vi "PI_GCS3_Configuration_Setup_FRF.vi"(0 "System no.":i32=1 min=1 step=1, 1 "Conn. Axes":string[](array[string]), 3 "Reference mode":enum16{"Do not reference", "Reference switch"}[](array[ring]), 5 "error in":errorcluster, 7 "Stop refnum":refnum<vi>) -> (19 "error out":errorcluster)   [LabVIEW 2020]
doc: "Select axes which reference mode is not \"Do not reference\" and waits until referenced with FRF. Former GCS 2.0 commands FPL/FNL are not supported any more.\n\nWarning: Do not use this VI outside the GCS 3.0 Configuration Setup."
uses:
  Special command.llb/ModeOfOperation.ctl
panel:
  # "Select axes which reference mode is not\n\"Do not reference\" and waits until referenced\nwith FRF. Former GCS 2.0 commands FPL/FNL\nare not supported any more.\n\nWarning: Do not use this VI outside the\nGCS 3.0 Configuration Setup."
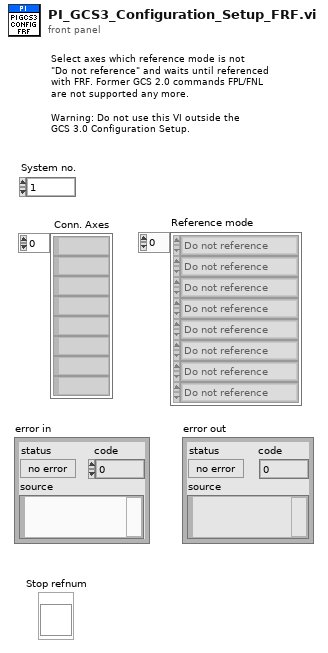
[diagram p1: front panel]
types:
  T1 = typedef "ModeOfOperation.ctl" = enum16{"Open", "Open-Loop Position", "Closed-Loop Position", "Open-Loop Velocity", "Closed-Loop Velocity", "Open-Loop Force", "Closed-Loop Force", "Step Operation"}
  T2 = typedef "Status.ctl" = cluster{"Element":string, "Status bits":bool[]}
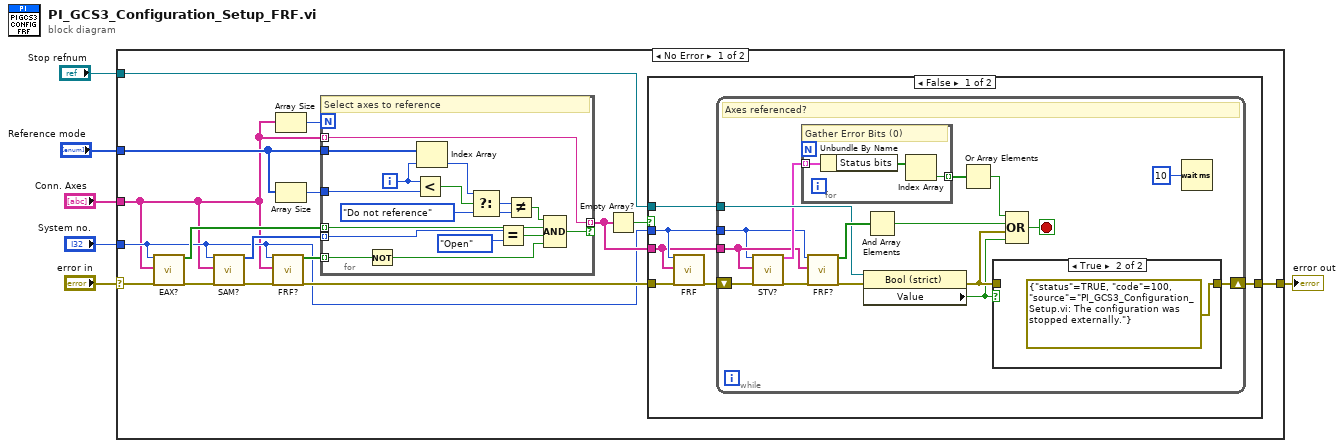
[diagram p0: block diagram]
diagram:
  n1 = case shown="No Error" "error in" {
    selector: "error in" -> [w16 w67]
    tunnel: [w22 w67] -> w5
    tunnel: "Conn. Axes" -> [w7 _]
    tunnel: "System no." -> [w8 _]
    tunnel: "Reference mode" -> [w17 _]
    tunnel: "Stop refnum" -> [w20 _]
    frame No Error {
      n2 = call "EAX?.vi"("System no."=w8, "Axes to query"=w7, "error in"=w16) -> ("Axes enabled status"=w12:bool[], "error out"=w15:errorcluster)  [unwired: 15 in]
      n3 = call "SAM?.vi"("System no."=w8, "Axis"=w7, "error in"=w15) -> ("Mode of Operations"=w13:T1[], "error out"=w11:errorcluster)  [unwired: 15 in]
      n4 = call "FRF?.vi"("System no."=w8, "Axes to query"=w7, "error in"=w11) -> ("Referenced?"=w9:bool[], "error out"=w10:errorcluster)  [unwired: 15 in]
      n5 = Array Size(array=w7) -> (size(s)=w18:i32)
      n6 = Array Size(array=w17) -> (size(s)=w19:i32)
      n7 = for {
        N: w18 -> [_]
        tunnel: w17 -> [w36]
        tunnel: w19 -> [w38]
        tunnel: w7 -> [w33] mode=indexing
        tunnel: [w33] -> w14 mode=indexing if=w29
        tunnel: w13 -> [w26] mode=indexing
        tunnel: w12 -> [w25] mode=indexing
        tunnel: w9 -> [w24] mode=indexing
        i -> [w35]
        w27 = enum16{"Do not reference", "Reference switch"}."Do not reference" ("element")
        # "Select axes to reference"
        n8 = Not(x=w24) -> (.not. x?=w23:bool)
        n9 = Less?(x=w35, y=w38) -> (x < y?=w37:bool)
        n10 = Index Array(array=w36, index=w35) -> (element=w34:enum16{"Do not reference", "Reference switch"})
        n11 = Select(t=w34, s=w37, f=w27) -> (s? t:f=w28:enum16{"Do not reference", "Reference switch"})
        n12 = Equal?(x=w26, y=ModeOfOperation."Open" ("Drive State")) -> (x = y?=w32:bool)
        n13 = Not Equal?(x=w28, y=w27) -> (x != y?=w31:bool)
        n14 = Compound Arithmetic op=AND(w31, w25, w32, w23) -> (w29:bool)
      }
      n15 = Empty Array?(array=w14) -> (empty?=w21:bool)
      n16 = case shown="False" w21 {
        tunnel: [w44 w66] -> w22
        tunnel: w10 -> [w43 w66]
        tunnel: w8 -> [w41 _]
        tunnel: w14 -> [w40 _]
        tunnel: w20 -> [w39 _]
        frame False {
          n17 = call "FRF.vi"("System no."=w41, "Affected axes"=w40, "error in"=w43) -> ("error out"=w42:errorcluster)  [unwired: 16 in]
          n18 = while {
            shift-right: [w56] -> w44
            shift-left: w42 -> [w50]
            tunnel: w41 -> [w47]
            tunnel: w40 -> [w48]
            tunnel: w39 -> [w58]
            stop <- w52 stop-if-true
            # "Axes referenced?"
            n19 = call "STV?.vi"("System no."=w47, "Status Type"=w48, "error in"=w50) -> ("Status Array"=w51:T2[], "error out"=w49:errorcluster)  [unwired: 15 in]
            n20 = for {
              tunnel: w51 -> [w62] mode=indexing
              tunnel: [w61] -> w46 mode=indexing
              # "Gather Error Bits (0)"
              n21 = Unbundle By Name(w62) -> ("Status bits"=w63:bool[])
              n22 = Index Array(array=w63) -> (element=w61:bool)  [unwired: 1 in]
            }
            n23 = call "FRF?.vi"("System no."=w47, "Axes to query"=w48, "error in"=w49) -> ("Referenced?"=w60:bool[], "error out"=w59:errorcluster)  [unwired: 15 in]
            n24 = property class="Bool (strict)"(reference=w58, error in=w59) -> (error out=w54:errorcluster, "Value"=w53:bool)  [unwired: 1 out]
            n25 = And Array Elements(Boolean array=w60) -> (logical AND=w55:bool)
            n26 = Or Array Elements(Boolean array=w46) -> (logical OR=w45:bool)
            n27 = case shown="True" w53 {
              tunnel: [w64 errorcluster {"status"=TRUE, "code"=100, "source"="PI_GCS3_Configuration_Setup.vi: The configuration was stopped externally."} ("error out")] -> w56
              tunnel: w54 -> [w64 _]
              frame False {
              }
              frame True {
              }
            }
            n28 = Compound Arithmetic op=OR(w45, w55, w54, w53) -> (w52:bool)
            n29 = Wait (ms)(milliseconds to wait=u32 10) -> ()  [unwired: 1 out]
          }
        }
        frame True {
        }
      }
    }
    frame Error {
    }
  }
  "error out" <- w5
